vi "pf_Config_MultipleROI_and_Grab.vi"() -> ()   [LabVIEW 2012]
uses:
  <userlib>/Photonfocus Toolkit/_Public/SubVIs/pf_Set_Camera_Property_Float.vi
  <userlib>/Photonfocus Toolkit/_Public/SubVIs/pf_Set_Camera_Property_Bool.vi
  <userlib>/Photonfocus Toolkit/_Public/SubVIs/pf_Set_Camera_Property_Int.vi
  <userlib>/Photonfocus Toolkit/Photonfocus_Toolkit.lvlib
panel:
  in  "stop":bool
  in  "Tab Control":enum32{"Instructions", "image"}(tab)
  in  "Interface Name":string="img0::0||port0"
  out "Image":T1(plugin-control)
  # "1 - Open MAX and specify the correct .icd file."
  # "2 - Get the interface name from MAX (e.g: \"imag0\") and write it in the following text field. \n\n3 - Add \"::\" and the Port number showed in MAX.\n\n4 - Add \"||\" and the port name showed in PFRemote."
  # "::"
  # "||port0"
  # "Example:   img0::0||port0"
  # "5 - Close MAX before start grabbing"
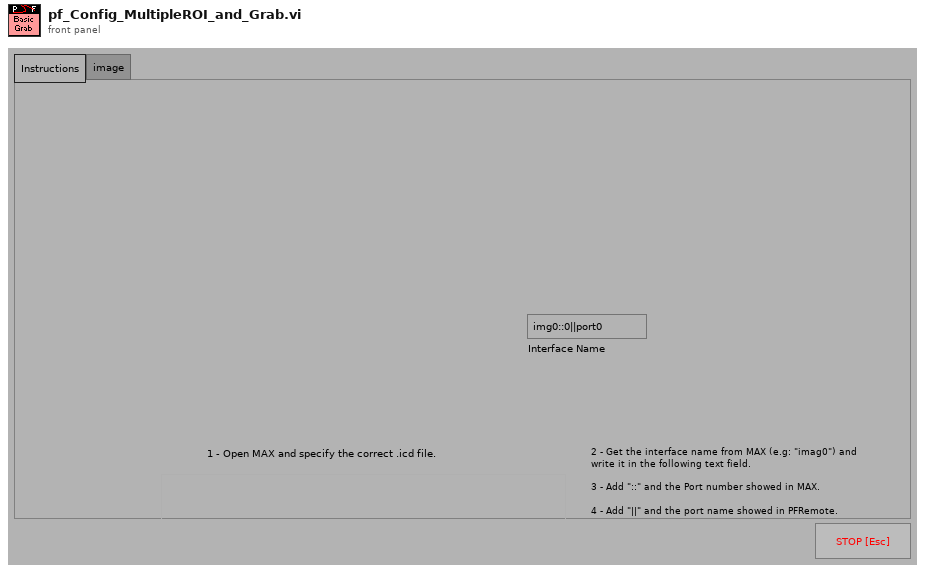
[diagram p1: front panel]
types:
  T1 = typedef "IMAQ Image.ctl" = refnum<image>
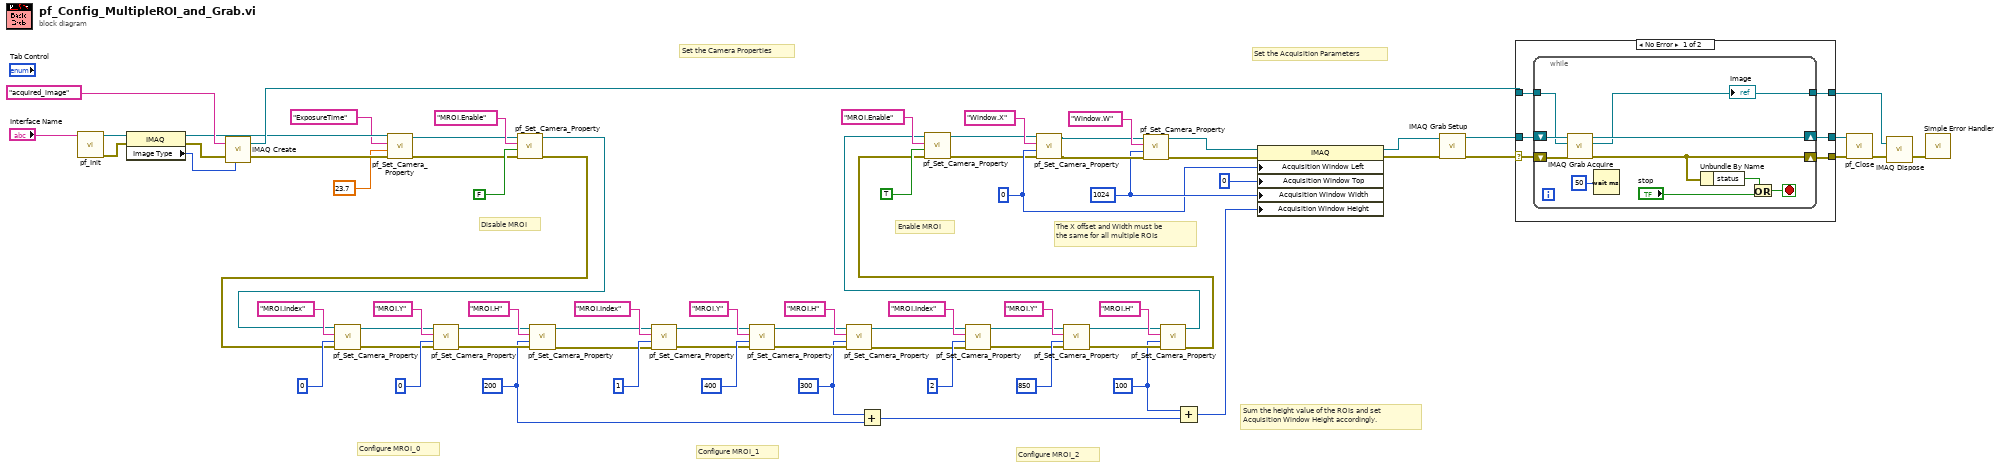
[diagram p0: block diagram]
diagram:
  w14 = u32 100 ("milliseconds to wait")
  w16 = u32 300 ("milliseconds to wait")
  w17 = u32 200 ("milliseconds to wait")
  w30 = u32 1024 ("milliseconds to wait")
  w29 = u32 0 ("milliseconds to wait")
  # "The X offset and Width must be \nthe same for all multiple ROIs"
  # "Set the Acquisition Parameters"
  # "Set the Camera Properties"
  # "Enable MROI"
  # "Sum the height value of the ROIs and set \nAcquisition Window Height accordingly."
  # "Configure MROI_2"
  # "Configure MROI_1"
  # "Configure MROI_0"
  # "Disable MROI"
  n1 = call <userlib>:"pf_Init.vi"("Interface Name"="Interface Name") -> ("error out"=w70:errorcluster, "IMAQ Session out"=w71:refnum<k11>)  [unwired: 2 in, 7 out]
  n2 = property class="IMAQ"(reference=w71, error in=w70) -> (reference out=w62:refnum<k11>, error out=w76:errorcluster, "Image Type"=w77:u32)
  n3 = call "IMAQ Create"("Image Name"="acquired_image", "Image Type"=w77, "error in (no error)"=w76) -> ("New Image"=w64:T1, "error out"=w63:errorcluster)  [unwired: 1 in, 1 out]
  n4 = call-poly <userlib>:"pf_Set_Camera_Property.vi"("error in (no error)"=w63, "Property Value"=23.7 ("milliseconds to wait"), "Property Name"="ExposureTime" ("Image Name"), "IMAQ Session in"=w62) -> ("error out"=w9:errorcluster, "IMAQ Session out"=w10:refnum<k11>)  [unwired: 5 in, 1 out]
  n5 = call-poly <userlib>:"pf_Set_Camera_Property.vi"("error in (no error)"=w9, "Property Value"=FALSE, "Property Name"="MROI.Enable" ("Image Name"), "IMAQ Session in"=w10) -> ("error out"=w8:errorcluster, "IMAQ Session out"=w7:refnum<k11>)  [unwired: 5 in, 1 out]
  n6 = call-poly <userlib>:"pf_Set_Camera_Property.vi"("error in (no error)"=w8, "Property Value"=u32 0 ("milliseconds to wait"), "Property Name"="MROI.Index" ("Image Name"), "IMAQ Session in"=w7) -> ("error out"=w46:errorcluster, "IMAQ Session out"=w45:refnum<k11>)  [unwired: 5 in, 1 out]
  n7 = call-poly <userlib>:"pf_Set_Camera_Property.vi"("error in (no error)"=w46, "Property Value"=u32 0 ("milliseconds to wait"), "Property Name"="MROI.Y" ("Image Name"), "IMAQ Session in"=w45) -> ("error out"=w42:errorcluster, "IMAQ Session out"=w43:refnum<k11>)  [unwired: 5 in, 1 out]
  n8 = call-poly <userlib>:"pf_Set_Camera_Property.vi"("error in (no error)"=w42, "Property Value"=w17, "Property Name"="MROI.H" ("Image Name"), "IMAQ Session in"=w43) -> ("error out"=w31:errorcluster, "IMAQ Session out"=w32:refnum<k11>)  [unwired: 5 in, 1 out]
  n9 = call-poly <userlib>:"pf_Set_Camera_Property.vi"("error in (no error)"=w31, "Property Value"=u32 1 ("milliseconds to wait"), "Property Name"="MROI.Index" ("Image Name"), "IMAQ Session in"=w32) -> ("error out"=w37:errorcluster, "IMAQ Session out"=w36:refnum<k11>)  [unwired: 5 in, 1 out]
  n10 = call-poly <userlib>:"pf_Set_Camera_Property.vi"("error in (no error)"=w37, "Property Value"=u32 400 ("milliseconds to wait"), "Property Name"="MROI.Y" ("Image Name"), "IMAQ Session in"=w36) -> ("error out"=w33:errorcluster, "IMAQ Session out"=w34:refnum<k11>)  [unwired: 5 in, 1 out]
  n11 = call-poly <userlib>:"pf_Set_Camera_Property.vi"("error in (no error)"=w33, "Property Value"=w16, "Property Name"="MROI.H" ("Image Name"), "IMAQ Session in"=w34) -> ("error out"=w18:errorcluster, "IMAQ Session out"=w19:refnum<k11>)  [unwired: 5 in, 1 out]
  n12 = Add(x=w16, y=w17) -> (x+y=w15:u32)
  n13 = call-poly <userlib>:"pf_Set_Camera_Property.vi"("error in (no error)"=w18, "Property Value"=u32 2 ("milliseconds to wait"), "Property Name"="MROI.Index" ("Image Name"), "IMAQ Session in"=w19) -> ("error out"=w24:errorcluster, "IMAQ Session out"=w23:refnum<k11>)  [unwired: 5 in, 1 out]
  n14 = call-poly <userlib>:"pf_Set_Camera_Property.vi"("error in (no error)"=w24, "Property Value"=u32 850 ("milliseconds to wait"), "Property Name"="MROI.Y" ("Image Name"), "IMAQ Session in"=w23) -> ("error out"=w20:errorcluster, "IMAQ Session out"=w21:refnum<k11>)  [unwired: 5 in, 1 out]
  n15 = call-poly <userlib>:"pf_Set_Camera_Property.vi"("error in (no error)"=w20, "Property Value"=w14, "Property Name"="MROI.H" ("Image Name"), "IMAQ Session in"=w21) -> ("error out"=w2:errorcluster, "IMAQ Session out"=w1:refnum<k11>)  [unwired: 5 in, 1 out]
  n16 = call-poly <userlib>:"pf_Set_Camera_Property.vi"("error in (no error)"=w2, "Property Value"=TRUE, "Property Name"="MROI.Enable" ("Image Name"), "IMAQ Session in"=w1) -> ("error out"=w3:errorcluster, "IMAQ Session out"=w4:refnum<k11>)  [unwired: 5 in, 1 out]
  n17 = call-poly <userlib>:"pf_Set_Camera_Property.vi"("error in (no error)"=w3, "Property Value"=w29, "Property Name"="Window.X" ("Image Name"), "IMAQ Session in"=w4) -> ("error out"=w54:errorcluster, "IMAQ Session out"=w53:refnum<k11>)  [unwired: 5 in, 1 out]
  n18 = call-poly <userlib>:"pf_Set_Camera_Property.vi"("error in (no error)"=w54, "Property Value"=w30, "Property Name"="Window.W" ("Image Name"), "IMAQ Session in"=w53) -> ("error out"=w52:errorcluster, "IMAQ Session out"=w51:refnum<k11>)  [unwired: 5 in, 1 out]
  n19 = Add(x=w14, y=w15) -> (x+y=w13:u32)
  n20 = property on="Property Node" class="IMAQ"(reference=w51, error in=w52, "Acquisition Window Left"=w29, "Acquisition Window Top"=u32 0 ("milliseconds to wait"), "Acquisition Window Width"=w30, "Acquisition Window Height"=w13) -> (reference out=w56:refnum<k11>, error out=w57:errorcluster)
  n21 = call <vilib>:"IMAQ Grab Setup.vi"("error in (no error)"=w57, "IMAQ Session In"=w56) -> ("error out"=w65:errorcluster, "IMAQ Session Out"=w67:refnum<k11>)  [unwired: 8 out]
  n22 = case shown="No Error" w65 {
    selector: w65 -> [w80 w96]
    tunnel: [w78 w96] -> w69
    tunnel: w64 -> [w83 w95]
    tunnel: [w82 w95] -> w73
    tunnel: w67 -> [w81 w94]
    tunnel: [w79 w94] -> w66
    frame No Error {
      n23 = while {
        tunnel: w83 -> [w85]
        tunnel: [w86] -> w82
        shift-right: [w84] -> w78
        shift-left: w80 -> [w88]
        shift-right: [w87] -> w79
        shift-left: w81 -> [w89]
        stop <- w90 stop-if-true
        n24 = call <vilib>:"IMAQ Grab Acquire.vi"("error in (no error)"=w88, "Image In"=w85, "IMAQ Session In"=w89) -> ("error out"=w84:errorcluster, "Image Out"=w86:T1, "IMAQ Session Out"=w87:refnum<k11>)  [unwired: 1 in, 5 out]
        "Image" <- w86
        n25 = Wait (ms)(milliseconds to wait=u32 50) -> ()  [unwired: 1 out]
        n26 = Unbundle By Name(w84) -> ("status"=w91:bool)
        n27 = Or(x=w91, y="stop") -> (x .or. y?=w90:bool)
      }
    }
    frame Error {
    }
  }
  n28 = call <userlib>:"pf_Close.vi"("error in (no error)"=w69, "IMAQ Session in"=w66) -> ("error out"=w68:errorcluster)  [unwired: 9 out]
  n29 = call "IMAQ Dispose"("Image"=w73, "error in (no error)"=w68) -> ("error out"=w75:errorcluster)  [unwired: 1 in, 3 out]
  n30 = call <vilib>:"Simple Error Handler.vi"("error in (no error)"=w75) -> ()  [unwired: 1 in, 8 out]
